vi "Write Value.vi"(8 "error in (no error)":errorcluster, 10 "Value":waveform(dbl)[](array[waveform]), 11 "Const_WFM in":refnum<class "Const_WFM_1D.lvclass">) -> (0 "error out":errorcluster, 3 "Const_WFM out":refnum<class "Const_WFM_1D.lvclass">)   [LabVIEW 2021, in "Const_WFM_1D.lvclass"]
uses:
  Const_WFM_1D.lvclass
  Const_WFM_1D.lvclass/Const_WFM_1D.ctl
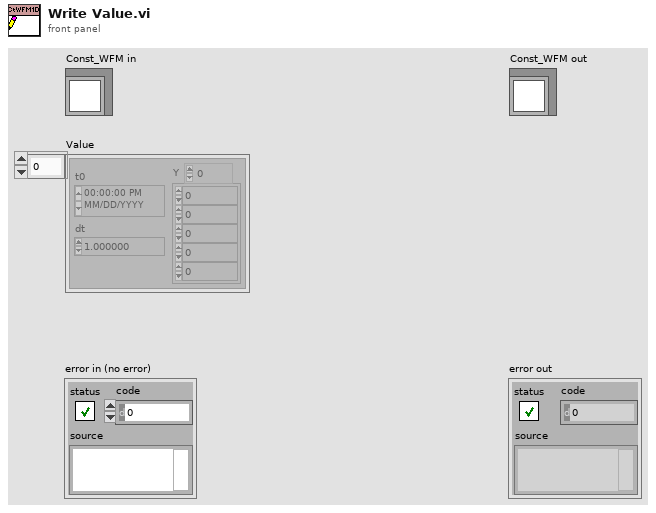
[diagram p1: front panel]
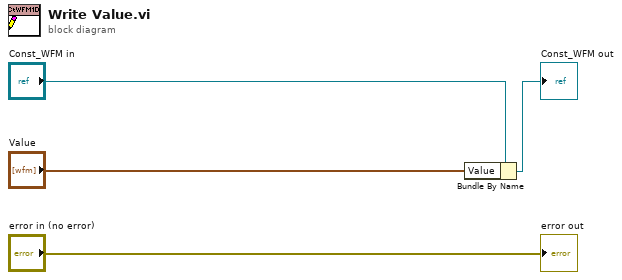
[diagram p0: block diagram]
diagram:
  n1 = Bundle By Name(cluster="Const_WFM in", "Value"="Value") -> (→"Const_WFM out":refnum<class "Const_WFM_1D.lvclass">)
  "error out" <- "error in (no error)"
